vi "SetEvent.vi"(8 "error in (no error)":errorcluster, 10 "event":string, 11 "PredictiveMaintenance in":refnum<class "PredictiveMaintenance.lvclass">) -> (0 "error out":errorcluster, 3 "PredictiveMaintenance out":refnum<class "PredictiveMaintenance.lvclass">)   [LabVIEW 2019, in "PredictiveMaintenance.lvlib" / "PredictiveMaintenance.lvclass"]
uses:
  PredictiveMaintenance.lvclass
  PredictiveMaintenance.lvclass/PredictiveMaintenance.ctl
  typedefs/EventData.ctl
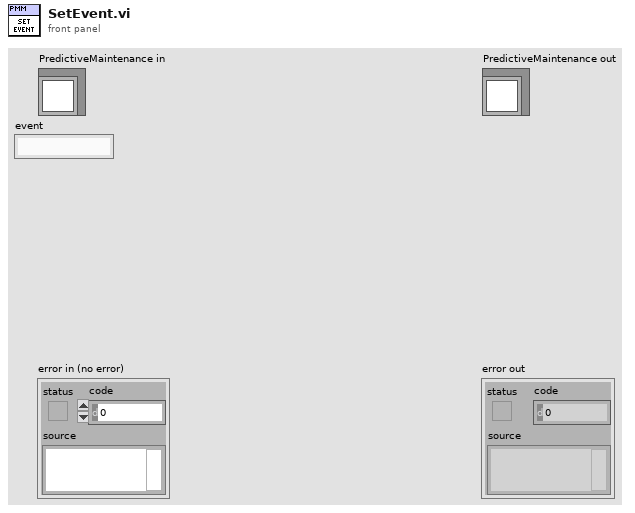
[diagram p1: front panel]
types:
  T1 = typedef "PredictiveMaintenance.lvlib/PredictiveMaintenance.lvclass/EventData.ctl" = cluster{"event":string, "curr_val":dbl, "warn_limit":dbl, "err_limit":dbl}
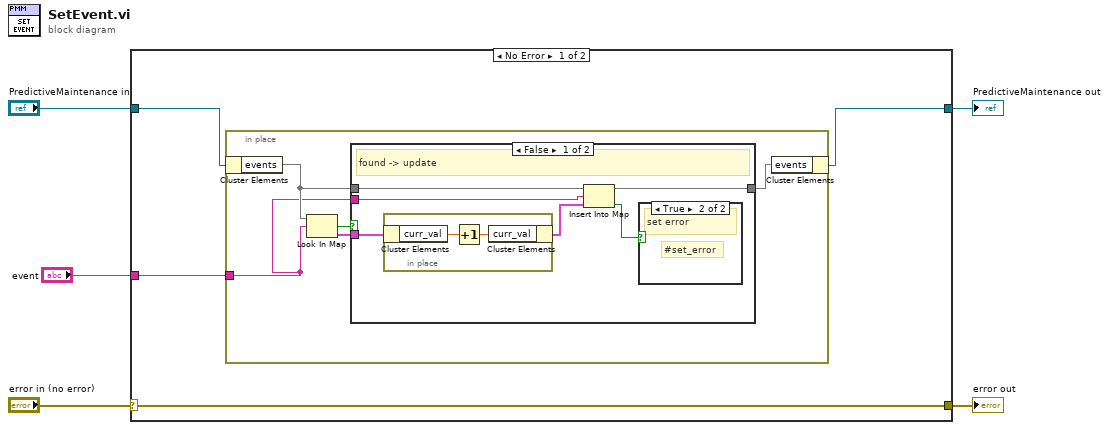
[diagram p0: block diagram]
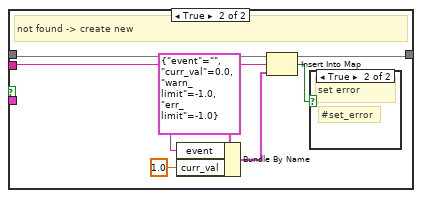
[diagram p3: hidden frame]
diagram:
  n1 = case shown="No Error" "error in (no error)" {
    selector: "error in (no error)" -> [w9 w31]
    tunnel: [w9 w31] -> w4
    tunnel: [w7 w30] -> w2
    tunnel: "PredictiveMaintenance in" -> [w8 w30]
    tunnel: "event" -> [w6 _]
    frame No Error {
      n2 = in-place {
        in-place-border: w6 -> [w10]
        n3 = in-place-cluster #1(w8) -> ("events"=w13:map{string, T1})
        n4 = Look In Map(map=w13, key=w10) -> (key not found?=w14:bool, value=w12:T1)  [unwired: 1 in]
        n5 = case shown="False" w14 {
          tunnel: w13 -> [w20 w29]
          tunnel: w12 -> [w18 _]
          tunnel: [w19 w28] -> w11
          tunnel: w10 -> [w16 w25]
          frame False {
            # "found -> update"
            n6 = in-place {
              n7 = in-place-cluster #2(w18) -> ("curr_val"=w22:dbl)
              n8 = Increment(x=w22) -> (x+1=w21:dbl)
              n9 = in-place-cluster #2("curr_val"=w21) -> (w17:T1)
            }
            n10 = Insert Into Map(map in=w20, key=w16, value=w17) -> (map out=w19:map{string, T1}, value unchanged?=w15:bool)  [unwired: 1 out]
            n11 = case shown="True" w15 {
              frame False {
              }
              frame True {
                # "#set_error"
                # "set error"
              }
            }
          }
          frame True {
            # "not found -> create new"
            n12 = Bundle By Name(cluster=T1 {"event"="", "curr_val"=0.0, "warn_limit"=-1.0, "err_limit"=-1.0} ("value"), "event"=w25, "curr_val"=1.0) -> (w26:T1)
            n13 = Insert Into Map(map in=w29, key=w25, value=w26) -> (map out=w28:map{string, T1}, key already included?=w23:bool)  [unwired: 1 out]
            n14 = case shown="True" w23 {
              frame False {
              }
              frame True {
                # "#set_error"
                # "set error"
              }
            }
          }
        }
        n15 = in-place-cluster #1("events"=w11) -> (w7:refnum<class "PredictiveMaintenance.lvclass">)
      }
    }
    frame Error {
    }
  }
  "error out" <- w4
  "PredictiveMaintenance out" <- w2
